vi "startUp.vi"(8 "error in (no error)":errorcluster, 11 "ScanCreator in":refnum<class "ScanCreator.lvclass">) -> (0 "error out":errorcluster, 3 "ScanCreator out":refnum<class "ScanCreator.lvclass">)   [LabVIEW 2009, in "Views.lvlib" / "ScriptEditor.lvlib" / "ScanCreator.lvclass"]
uses:
  ScanCreator.lvclass
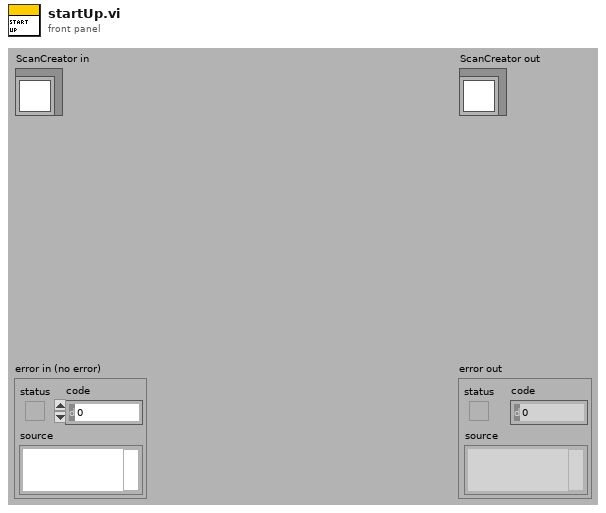
[diagram p1: front panel]
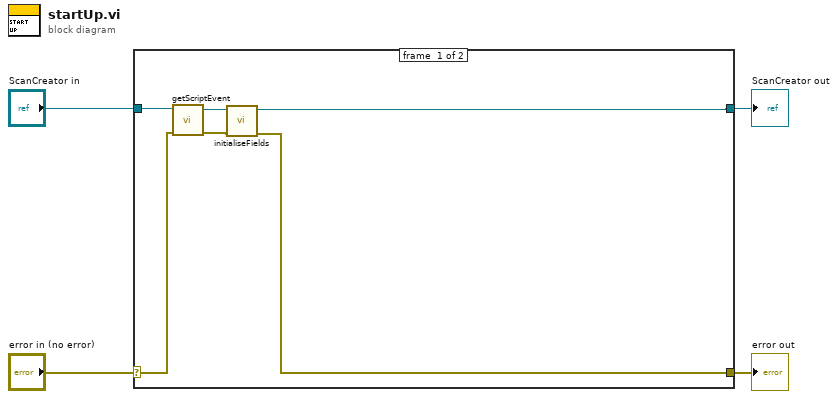
[diagram p0: block diagram]
diagram:
  n1 = case shown="No Error" "error in (no error)" {
    selector: "error in (no error)" -> [w6 w12]
    tunnel: [w5 w12] -> w3
    tunnel: [w7 w11] -> w1
    tunnel: "ScanCreator in" -> [w10 w11]
    frame #0 {
      n2 = call "getScriptEvent.vi"("error in (no error)"=w6, "ScanCreator in"=w10) -> ("error out"=w8:errorcluster, "ScanCreator out"=w9:refnum<class "ScanCreator.lvclass">)  [unwired: 8 in]
      n3 = call "initialiseFields.vi"("error in (no error)"=w8, "ScanCreator in"=w9) -> ("error out"=w5:errorcluster, "ScanCreator out"=w7:refnum<class "ScanCreator.lvclass">)  [unwired: 8 in]
    }
    frame #1 {
    }
  }
  "error out" <- w3
  "ScanCreator out" <- w1
